vi "teleop.vi"(10 "Match Info":T1={"Autonomous Elapsed Seconds"=0.0, "TeleOp Elapsed Seconds"=0.0, "Disabled Elapsed Seconds"=0.0, "Visited Autonomous"=FALSE, "Visited TeleOp"=FALSE, "Visited Disabled"=FALSE, "Autonomous Settings"={"Autonomous Style"=enum."Independent", "VI Refnum"=refnum}}, 11 "Call Context":T2) -> ()   [LabVIEW 2011]
doc: "This VI is called for each TeleOp packet received from the DS where the robot is not disabled. It is often used to read from the joysticks and update I/O or to update setpoints for timed control loops. It should complete and return within 20 milliseconds or it may miss DS packets."
uses:
  <vilib>/Rock Robotics/WPI/DriverStation/WPI_DriverStationDerivedRobotMode.ctl
  <vilib>/Rock Robotics/WPI/DriverStation/WPI_DriverStationMatch Info.ctl
  <vilib>/Rock Robotics/WPI/Relay/WPI_RelayValue.ctl
  <vilib>/Rock Robotics/WPI/Solenoid/WPI_SolenoidValue.ctl
  Robot Global Data.vi
  <vilib>/Rock Robotics/WPI/Solenoid/WPI_SolenoidSetEnum.vi
  <vilib>/Rock Robotics/WPI/RobotDrive/WPI_RobotDriveArcadeDrive_Standard(NoSaturation).vi
panel:
  in  "offset":dbl=2.0
  in  "shot delay":dbl=0.8
  in  "speedFactor":dbl=1.1
  in  "speedScaling":dbl=0.8
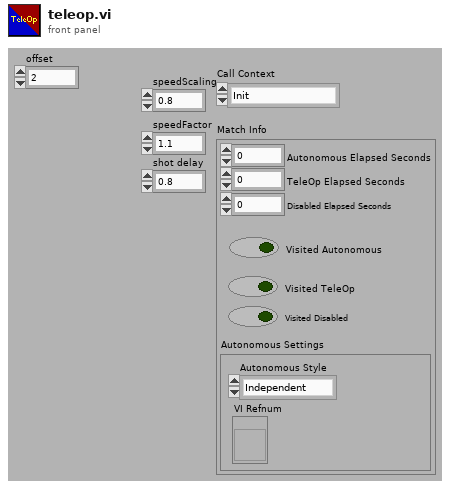
[diagram p1: front panel]
types:
  T1 = typedef "WPI_DriverStationMatch Info.ctl" = cluster{"Autonomous Elapsed Seconds":dbl, "TeleOp Elapsed Seconds":dbl, "Disabled Elapsed Seconds":dbl, "Visited Autonomous":bool, "Visited TeleOp":bool, "Visited Disabled":bool, "Autonomous Settings":cluster{"Autonomous Style":enum16{"Iterative", "Independent"}, "VI Refnum":refnum<vi>}}
  T2 = typedef "WPI_DriverStationDerivedRobotMode.ctl" = enum16{"Init", "Execute", "Stop"}
  T3 = typedef "WPI_SolenoidValue.ctl" = enum16{"Off", "On", "Forward", "Reverse"}
  T4 = typedef "WPI_RelayValue.ctl" = enum16{"Off", "On", "Forward", "Reverse"}
  T5 = typedef "WPI_RobotDriveDevRef.ctl" = cluster{"DevStatus":errorcluster, "Motors[]":T6[], "Square Inputs":bool, "Max Output":dbl, "Isochronous":bool}
  T6 = typedef "WPI_MotorControlDeviceRef.ctl" = cluster{"DeviceStatus":errorcluster, "Type":enum16{"PWM", "CAN"}, "PWM":cluster{"Digital Module":T7, "PWM Channel":T8, "DeadBand":T9}, "CAN":cluster{"Device Number":u8, "Control Mode":T10, "Semaphore":T11, "Max Vout":dbl}, "Invert":bool, "TransformRef":T12, "InvTransformRef":T12}
  T7 = typedef "FPGA_TypedefDigitalModule.ctl" = enum16{"Digital Module 1", "Digital Module 2"}
  T8 = typedef "FPGA_DIOPWMChannel.ctl" = enum8{"PWM 1", "PWM 2", "PWM 3", "PWM 4", "PWM 5", "PWM 6", "PWM 7", "PWM 8", "PWM 9", "PWM 10", "Invalid"}
  T9 = typedef "WPI_PWMDeadband.ctl" = cluster{"Name":string, "maxPositivePwm":i32, "minPositivePwm":i32, "centerPwm":i32, "maxNegativePwm":i32, "minNegativePwm":i32, "angularRange":u16}
  T10 = typedef "WPI_CANJaguar_ControlMode.ctl" = enum8{"Percent VBus", "Current", "Speed", "Position", "Voltage"}
  T11 = typedef "Semaphore RefNum" = refnum<k1>
  T12 = typedef "WPI_PWMTransform_ConPane.ctl" = refnum<vi>
  T13 = typedef "WPI_JoystickDevRef.ctl" = cluster{"Device":T14}
  T14 = typedef "WPI_JoystickDeviceEnum.ctl" = enum16{"USB 1", "USB 2", "USB 3", "USB 4", "Kinect 1", "Kinect 2"}
  T15 = typedef "WPI_JoystickButtonState.ctl" = cluster{"Button 1":bool, "Button 2":bool, "Button 3":bool, "Button 4":bool, "Button 5":bool, "Button 6":bool, "Button 7":bool, "Button 8":bool, "Button 9":bool, "Button 10":bool, "Button 11":bool, "Button 12":bool}
  T16 = cluster{"axis 1 (x)":dbl, "axis 2 (y)":dbl, "axis 3 (throttle)":dbl, "axis 4":dbl, "axis 5":dbl, "axis 6":dbl}
  T17 = typedef "WPI_RelayDevRef.ctl" = cluster{"DevStatus":errorcluster, "Relay Channel":T18, "Digital Module":T7, "Relay Direction":T19}
  T18 = typedef "FPGA_DIORelayChannel.ctl" = enum8{"Relay 1", "Relay 2", "Relay 3", "Relay 4", "Relay 5", "Relay 6", "Relay 7", "Relay 8", "Invalid"}
  T19 = typedef "WPI_RelayDirection.ctl" = enum16{"Both directions", "Forward only", "Reverse only"}
  T20 = typedef "WPI_SolenoidDevRef.ctl" = cluster{"DevStatus":errorcluster, "Solenoid Module":T21, "Forward Solenoid Channel":T22, "Reverse Solenoid Channel":T22}
  T21 = typedef "FPGA_TypedefSolenoidModule.ctl" = enum16{"Solenoid Module 1", "Solenoid Module 2"}
  T22 = typedef "WPI_SolenoidChannel.ctl" = enum8{"Solenoid 1", "Solenoid 2", "Solenoid 3", "Solenoid 4", "Solenoid 5", "Solenoid 6", "Solenoid 7", "Solenoid 8", "Invalid"}
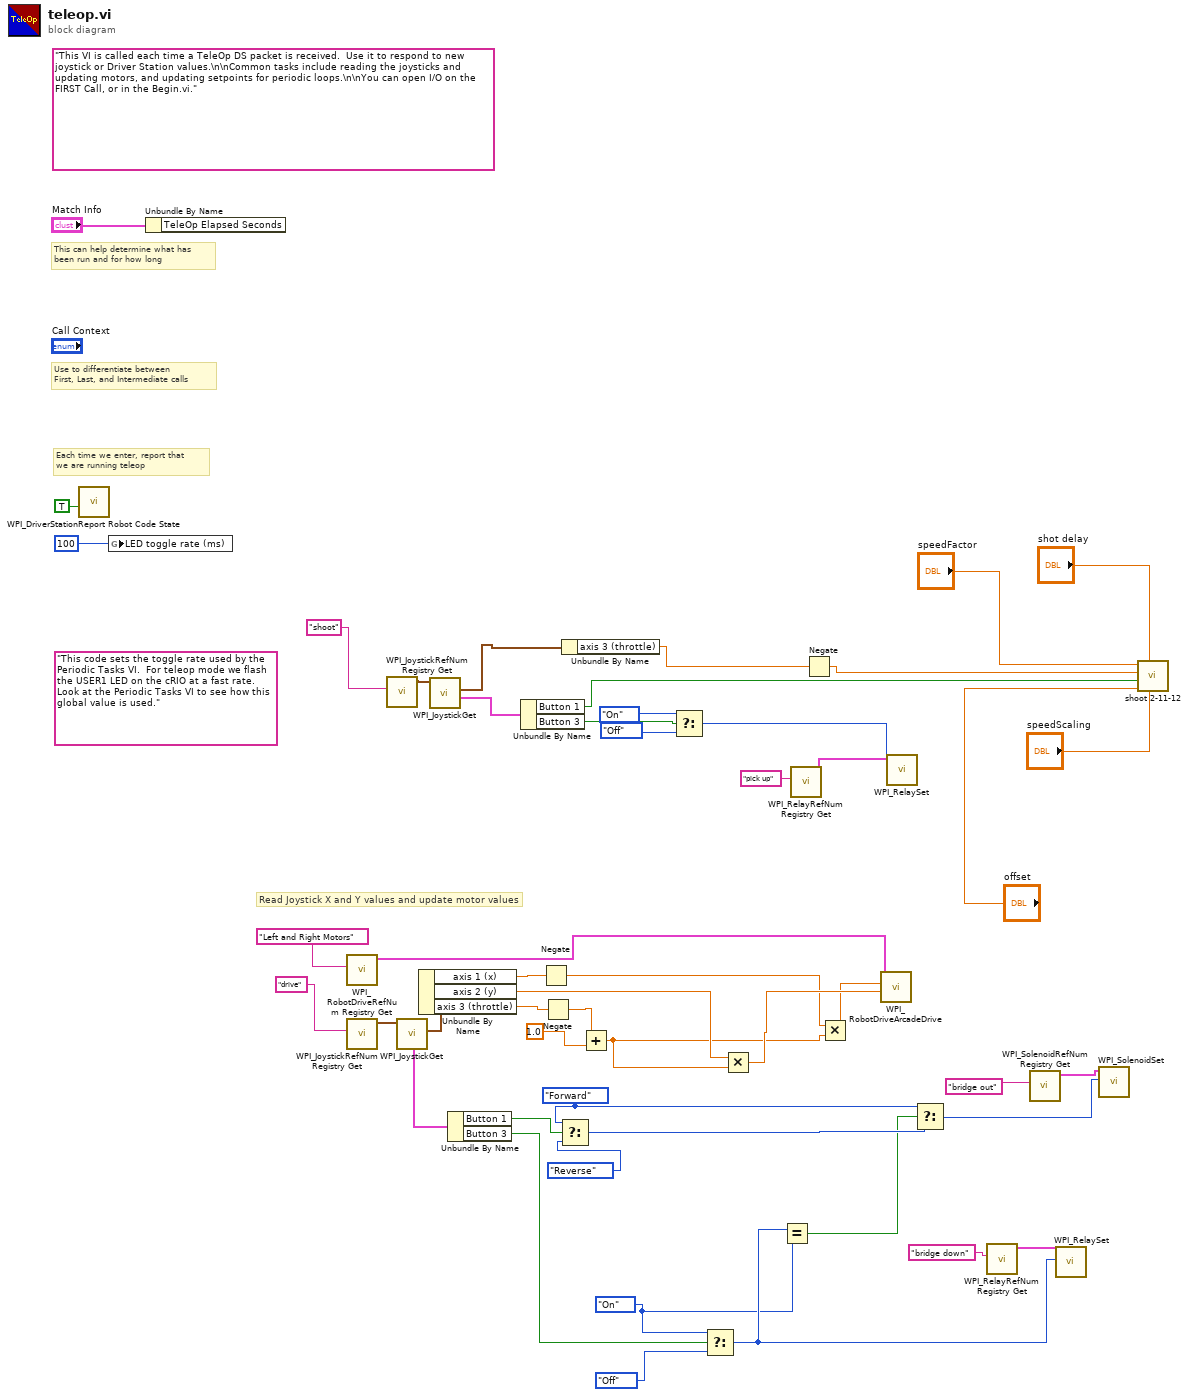
[diagram p0: block diagram]
diagram:
  w15 = WPI_SolenoidValue."On" ("Value")
  w11 = WPI_SolenoidValue."Forward" ("Value")
  (unwired) "This code sets the toggle rate used by the Periodic Tasks VI.  For teleop mode we flash the USER1 LED on the cRIO at a fast rate.  Look at the Periodic Tasks VI to see how this global value is used."
  (unwired) "This VI is called each time a TeleOp DS packet is received.  Use it to respond to new joystick or Driver Station values.\n\nCommon tasks include reading the joysticks and updating motors, and updating setpoints for periodic loops.\n\nYou can open I/O on the FIRST Call, or in the Begin.vi."
  # "Each time we enter, report that\nwe are running teleop"
  # "Use to differentiate between\nFirst, Last, and Intermediate calls"
  # "This can help determine what has\nbeen run and for how long"
  # "Read Joystick X and Y values and update motor values"
  n1 = call <vilib>:"WPI_DriverStationReport Robot Code State.vi"("TeleOp"=TRUE ("Autonomous")) -> ()  [unwired: 10 in, 1 out]
  n2 = global write "Robot Global Data.vi" "LED toggle rate (ms)"(u32 100 ("LED ms toggle rate")) -> ()
  n3 = Unbundle By Name("Match Info") -> ()  [unwired: 1 out]
  n4 = call <vilib>:"WPI_RobotDriveRefNum Registry Get.vi"("refnum name"="Left and Right Motors") -> ("RobotDriveDevRef"=w43:T5)  [unwired: 1 in, 9 out]
  n5 = call <vilib>:"WPI_JoystickRefNum Registry Get.vi"("refnum name"="drive") -> ("JoystickDevRef"=w46:T13)  [unwired: 1 in, 9 out]
  n6 = call <vilib>:"WPI_JoystickRefNum Registry Get.vi"("refnum name"="shoot") -> ("JoystickDevRef"=w40:T13)  [unwired: 1 in, 9 out]
  n7 = call <vilib>:"WPI_JoystickGet.vi"("JoystickDevRef"=w46) -> ("Buttons"=w29:T15, "Axes"=w47:T16)  [unwired: 1 in, 4 out]
  n8 = Unbundle By Name(w47) -> ("axis 1 (x)"=w42:dbl, "axis 2 (y)"=w7:dbl, "axis 3 (throttle)"=w2:dbl)
  n9 = call <vilib>:"WPI_JoystickGet.vi"("JoystickDevRef"=w40) -> ("Buttons"=w41:T15, "Axes"=w39:T16)  [unwired: 1 in, 4 out]
  n10 = Unbundle By Name(w29) -> ("Button 1"=w28:bool, "Button 3"=w25:bool)
  n11 = Unbundle By Name(w41) -> ("Button 1"=w38:bool, "Button 3"=w35:bool)
  n12 = Negate(x=w42) -> (-x=w6:dbl)
  n13 = Negate(x=w2) -> (-x=w1:dbl)
  n14 = Select(t=w11, s=w28, f=WPI_SolenoidValue."Reverse" ("Value")) -> (s? t:f=w14:T3)
  n15 = Unbundle By Name(w39) -> ("axis 3 (throttle)"=w10:dbl)
  n16 = Add(x=w1, y=1.0) -> (x+y=w3:dbl)
  n17 = Select(t=WPI_RelayValue."On" ("RelayValue"), s=w35, f=WPI_RelayValue."Off" ("RelayValue")) -> (s? t:f=w32:T4)
  n18 = Select(t=w15, s=w25, f=WPI_SolenoidValue."Off" ("Value")) -> (s? t:f=w16:T3)
  n19 = Multiply(x=w7, y=w3) -> (x*y=w8:dbl)
  n20 = Equal?(x=w16, y=w15) -> (x = y?=w12:bool)
  n21 = call <vilib>:"WPI_RelayRefNum Registry Get.vi"("refnum name"="pick up") -> ("RelayDevRef"=w36:T17)  [unwired: 9 in, 1 out]
  n22 = Negate(x=w10) -> (-x=w9:dbl)
  n23 = Multiply(x=w6, y=w3) -> (x*y=w5:dbl)
  n24 = call-poly <vilib>:"WPI_RobotDriveArcadeDrive.vi"("Y axis value"=w8, "X axis value"=w5, "RobotDriveDevRef"=w43) -> ()  [unwired: 7 in, 2 out]
  n25 = call <vilib>:"WPI_RelaySet.vi"("RelayValue"=w32, "RelayDevRef"=w36) -> ()  [unwired: 8 in, 2 out]
  n26 = Select(t=w11, s=w12, f=w14) -> (s? t:f=w13:T3)
  n27 = call <vilib>:"WPI_RelayRefNum Registry Get.vi"("refnum name"="bridge down") -> ("RelayDevRef"=w20:T17)  [unwired: 9 in, 1 out]
  n28 = call <vilib>:"WPI_SolenoidRefNum Registry Get.vi"("refnum name"="bridge out") -> ("SolenoidDevRef"=w30:T20)  [unwired: 9 in, 1 out]
  n29 = call <vilib>:"WPI_RelaySet.vi"("RelayValue"=w16, "RelayDevRef"=w20) -> ()  [unwired: 8 in, 2 out]
  n30 = call-poly <vilib>:"WPI_SolenoidSet.vi"("Value"=w13, "SolenoidDevRef"=w30) -> ()  [unwired: 8 in, 2 out]
  n31 = call "shoot 2-11-12.vi"("speedScaling"="speedScaling", "shot delay"="shot delay", "offset"="offset", "Button 1"=w38, "axis 3 (throttle)"=w9, "speedFactor"="speedFactor") -> ()  [unwired: 6 in]
